vi "Image_Acquire.vi"(0 "Queue Ref in":T3, 1 "Acquire Time":i32=100, 3 "Image Out":T1, 4 "Session In":T2, 5 "error in (no error)":errorcluster, 7 "Test Timing":bool) -> (6 "Loop Time Out":i64, 8 "error out":errorcluster)   [LabVIEW 2018]
uses:
  <vilib>/vision/Image Controls.llb/IMAQ Image.ctl
  <vilib>/userdefined/High Color/IMAQdx.ctl
  <vilib>/Platform/TimedLoop/XDataNode/timing_clust.ctl
  <vilib>/Platform/TimedLoop/XDataNode/nitl_modes.ctl
  <vilib>/Platform/TimedLoop/XDataNode/wakeup.ctl
  <vilib>/Platform/TimedLoop/XDataNode/XDataNode.xnode
  <vilib>/Platform/TimedLoop/XDataNode/XDNodeRunTimeDep.lvlib
  <vilib>/vision/driver/NI_Vision_Acquisition_Software.lvlib
panel:
  out "Image":T1(plugin-control)
  out "Global End Time":i64
  out "Iteration Duration":i64
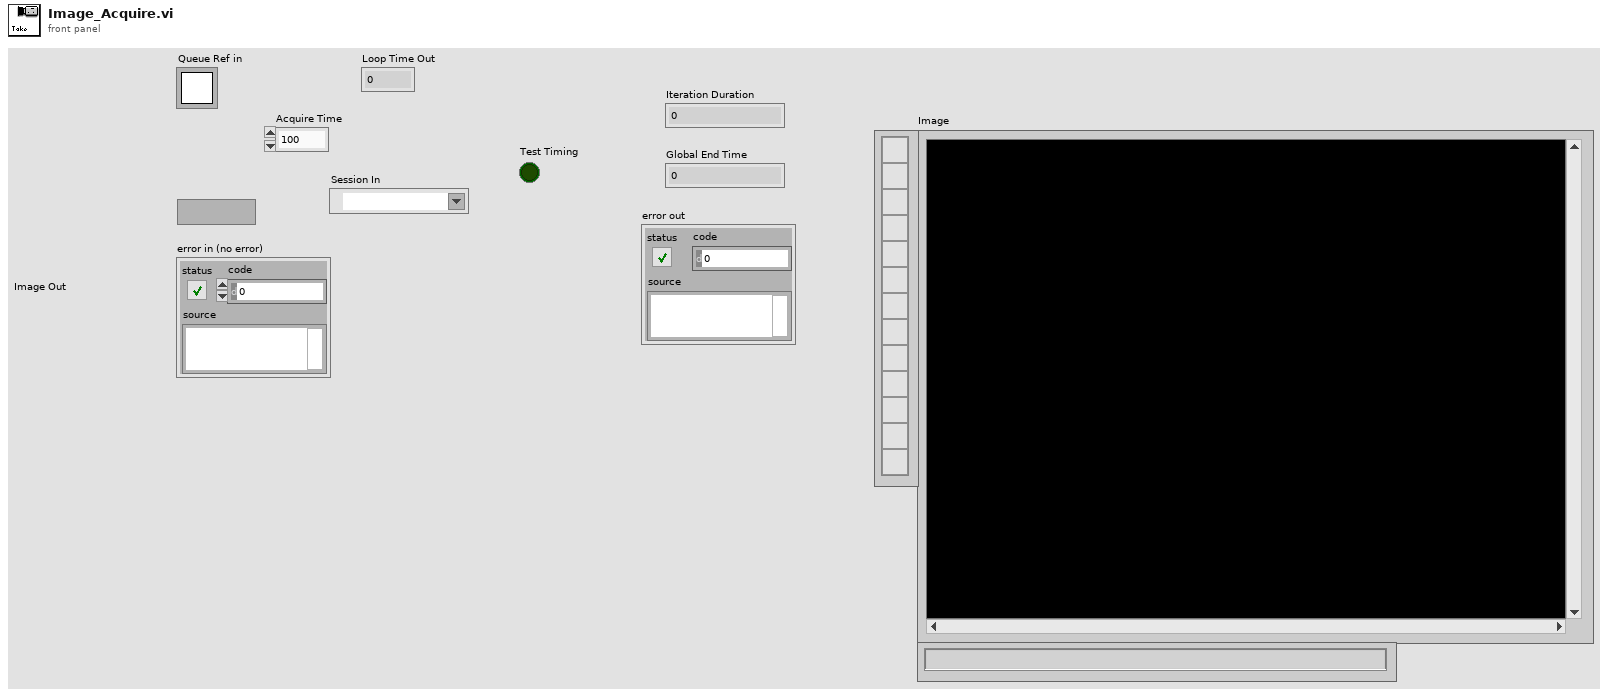
[diagram p1: front panel]
types:
  T1 = typedef "IMAQ Image.ctl" = refnum<image>
  T2 = typedef "IMAQdx.ctl" = refnum<k21>
  T3 = typedef "Queue RefNum" = refnum<k1>
  T4 = typedef "XDNodeRunTimeDep.lvlib/timing_clust.ctl" = cluster{"Expected End [f-1]":u64, "Actual End [f-1]":u64, "Finished Late? [f-1]":bool, "Expected End [i-1]":u64, "Actual End [i-1]":u64, "Finished Late? [i-1]":bool, "Expected Start [i]":u64, "Actual Start [i]":u64, "Expected Start [f]":u64, "Actual Start [f]":u64, "Source Name":string, "Structure Name":string, "Period":i64, "Deadline":i64, "Offset":i64, "Start":i64, "Priority":i32, "Timeout":i32, "Mode":T5, "Wakeup Reason":T6, "Error":errorcluster, "Source Type":string, "Secondary Source Type":string, "Global End Time":u64, "Global Start Time":u64, "Frame Duration":u64, "Iteration Duration":u64, "Assigned CPU":i32, "I/O Scan Engine Mode":u32}
  T5 = typedef "XDNodeRunTimeDep.lvlib/nitl_modes.ctl" = enum32{"No Change", "Process missed periods, maintain original phase", "Discard missed periods, maintain original phase", "Process missed periods, ignore original phase", "Discard missed periods, ignore original phase"}
  T6 = typedef "XDNodeRunTimeDep.lvlib/wakeup.ctl" = enum32{"Normal", "Aborted", "Asynchronous wakeup", "Timing source error", "Timed loop error", "Timeout"}
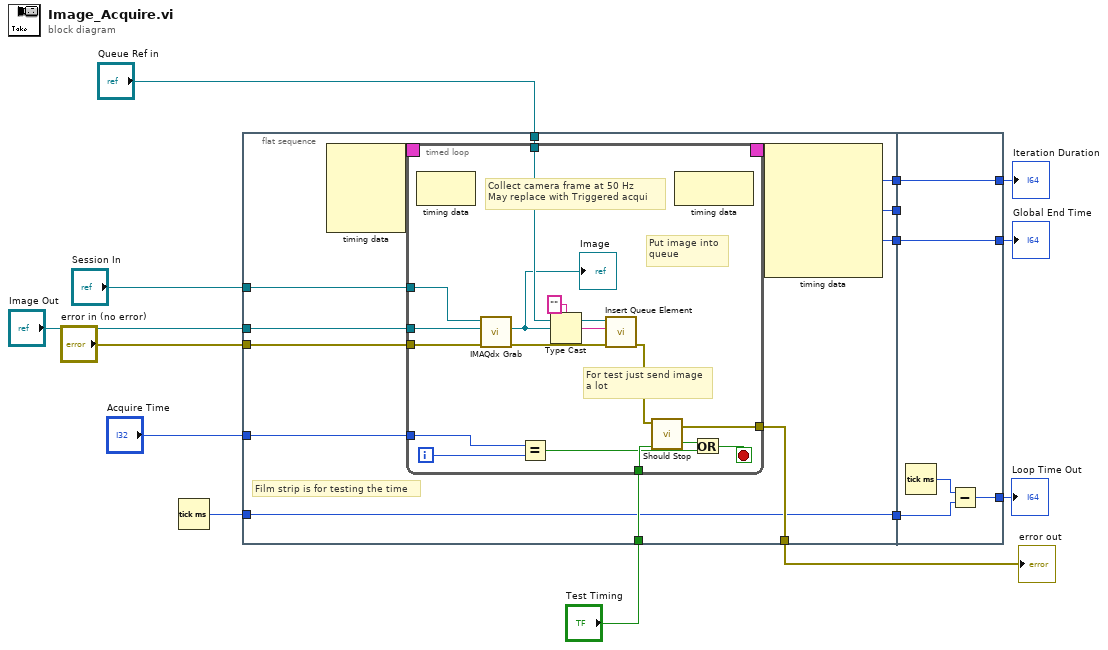
[diagram p0: block diagram]
diagram:
  n1 = Tick Count (ms)() -> (millisecond timer value=w1:u32)
  n2 = flat-sequence {
    tunnel: "error in (no error)" -> [w26]
    tunnel: "Image Out" -> [w25]
    tunnel: "Queue Ref in" -> [w24]
    tunnel: "Test Timing" -> [w23]
    tunnel: [w22] -> w11
    tunnel: [w21] -> w10
    tunnel: [w20] -> w8
    tunnel: [w19] -> w6
    tunnel: "Acquire Time" -> [w18]
    tunnel: "Session In" -> [w17]
    tunnel: [w16] -> w2
    tunnel: w1 -> [w16]
    tunnel: [w55] -> w9
    tunnel: w10 -> [w55]
    tunnel: [w56] -> w7
    tunnel: w8 -> [w56]
    tunnel: w6 -> [_]
    tunnel: [w52] -> w5
    tunnel: w2 -> [w53]
    frame #0 {
      # "Film strip is for testing the time"
      n3 = node-c288() -> (w28:T4)  [unwired: 4 in]
      n4 = timed-loop "Timed Loop" {
        timing: w28 -> [_]
        timing-out: [_] -> w27
        tunnel: w24 -> [w44]
        tunnel: [w42] -> w22
        tunnel: w26 -> [w33]
        tunnel: w25 -> [w31]
        tunnel: w23 -> [w39]
        tunnel: w18 -> [w38]
        tunnel: w17 -> [w32]
        i -> [w37]
        stop <- w35 stop-if-true
        # "Put image into\nqueue"
        # "For test just send image\na lot"
        # "Collect camera frame at 50 Hz\nMay replace with Triggered acqui"
        n5 = node-c288() -> ()  [unwired: 1 in, 1 out]
        n6 = call <vilib>:"IMAQdx Grab.vi"("error in"=w33, "Image In"=w31, "Session In"=w32) -> ("error out"=w30:errorcluster, "Image Out"=w29:T1)  [unwired: 1 in, 6 out]
        "Image" <- w29
        n7 = Equal?(x=w38, y=w37) -> (x = y?=w34:bool)
        n8 = Type Cast(type="", x=w29) -> (*(type *) &x=w40:string)
        n9 = call <vilib>:"Insert Queue Element.vi"("error in (no error)"=w30, "queue element"=w40, "queue"=w44) -> ("error out"=w43:errorcluster)  [unwired: 4 in, 2 out]
        n10 = call "Should Stop.vi"("error in 1"=w43, "Look at Stop Button"=w39) -> ("error out"=w42:errorcluster, "Stop"=w36:bool)  [unwired: 3 in]
        n11 = node-c288() -> ()  [unwired: 1 in, 1 out]
        n12 = Or(x=w36, y=w34) -> (x .or. y?=w35:bool)
      }
      n13 = node-c288(w27) -> (w21:i64, w19:i64, w20:i64)  [unwired: 4 out]
    }
    frame #1 {
      n14 = Tick Count (ms)() -> (millisecond timer value=w54:u32)
      n15 = Subtract(x=w54, y=w53) -> (x-y=w52:u32)
    }
  }
  "Loop Time Out" <- w5
  "error out" <- w11
  "Iteration Duration" <- w9
  "Global End Time" <- w7
